vi "SSL Log Reader.vi"(10 "Cluster 2":refnum<vi>, 11 "Cluster":T1={"file path (use dialog)"=path "E:/Media/2016-07-01_cmdragons_immortals.log", "size (in bytes)"=0, "offset (in bytes)"=0, "Slide"=0.0, "Play"=FALSE, "Time Stamp"=timestamp(0 s since 1904-01-01), "Playing"=FALSE} {"Time Stamp" format="%<%.3X %x>T"; "Slide" min=0 max=1 scale=0.0..1.0; "offset (in bytes)" format="%.3p"; "size (in bytes)" format="%.3p"}) -> (0 "error out":errorcluster, 1 "Cluster 3":T1={"file path (use dialog)"=path "E:/Media/2016-07-01_cmdragons_immortals.log", "size (in bytes)"=0, "offset (in bytes)"=0, "Slide"=0.0, "Play"=FALSE, "Time Stamp"=timestamp(0 s since 1904-01-01), "Playing"=FALSE} {"Time Stamp" format="%<%.3X %x>T"; "Slide" min=0 max=1 scale=0.0..1.0; "offset (in bytes)" format="%.3p"; "size (in bytes)" format="%.3p"}, 2 "channel 2":T2, 3 "Channel out":T2)   [LabVIEW 2017]
uses:
  <extravilib>/ChannelInstances/Stream-a[.](u8).lvlib
  <extravilib>/ChannelInstances/Stream-a[.](u8)/)Channel.ctl
  Control/File Player.ctl
panel:
  out "error out 2":errorcluster
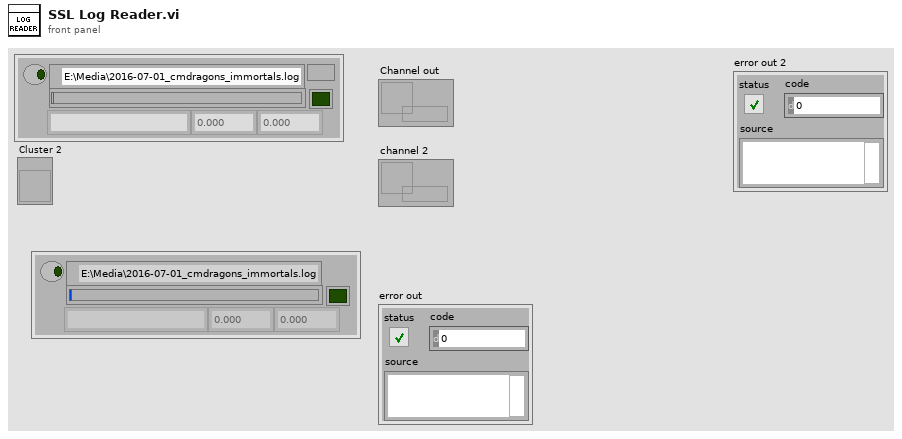
[diagram p1: front panel]
types:
  T1 = typedef "File Player.ctl" = cluster{"file path (use dialog)":path, "size (in bytes)":i64, "offset (in bytes)":i64, "Slide":sgl, "Play":bool, "Time Stamp":timestamp, "Playing":bool}
  T2 = typedef "Stream-a[.](u8).lvlib/)Channel.ctl" = refnum<queue>
  T3 = enum16{"open", "replace", "create", "open or create", "replace or create", "replace or create with confirmation"}
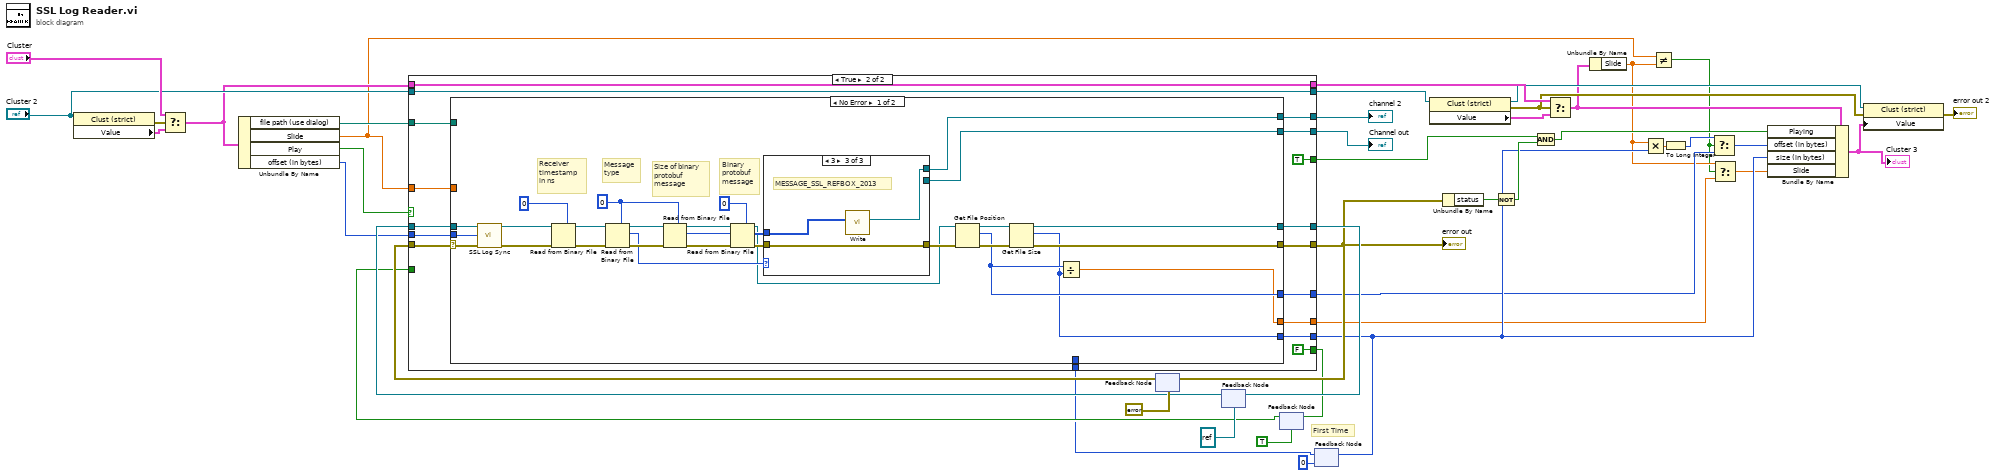
[diagram p0: block diagram]
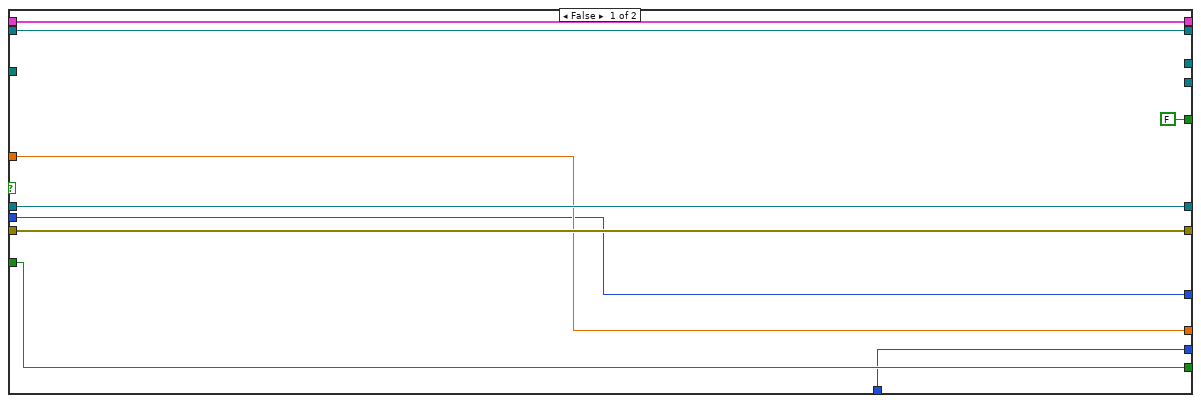
[diagram p2: hidden frame]
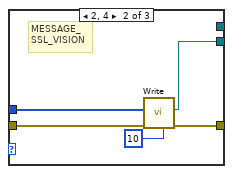
[diagram p4: hidden frame]
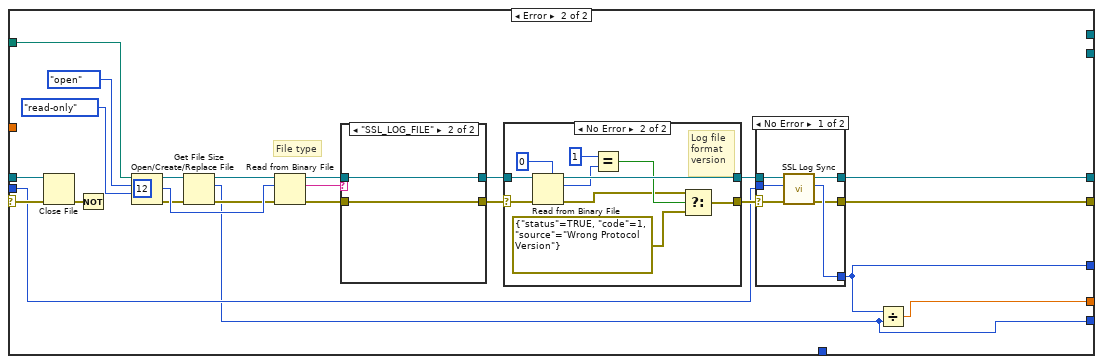
[diagram p5: hidden frame]
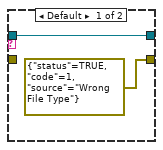
[diagram p7: hidden frame]
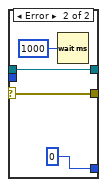
[diagram p8: hidden frame]
diagram:
  # "First Time"
  n1 = property on="Property Node" class="Clust (strict)"(reference="Cluster 2") -> (error out=w28:errorcluster, "Value"=w26:T1)  [unwired: 1 in, 1 out]
  n2 = Select(t="Cluster", s=w28, f=w26) -> (s? t:f=w19:T1)
  n3 = Unbundle By Name(w19) -> ("file path (use dialog)"=w25:path, "Slide"=w10:sgl, "Play"=w24:bool, "offset (in bytes)"=w13:i64)
  n4 = feedback #1(errorcluster {"status"=FALSE, "code"=0, "source"=""} ("error out")) -> (w39:errorcluster)
  n5 = feedback #2(refnum<file> refnum ("refnum out")) -> (w37:refnum<file>)
  n6 = feedback #3(TRUE) -> (w33:bool)
  n7 = feedback #4(i64 0 ("size (in bytes)")) -> (w30:i64)
  n8 = case shown="True" w24 {
    tunnel: [w44 w69] -> w7
    tunnel: w25 -> [_ w68]
    tunnel: [_ w67] -> w43
    tunnel: [_ w66] -> w42
    tunnel: w10 -> [w45 w63]
    tunnel: [w51 w65] -> w36
    tunnel: w39 -> [w51 w61]
    tunnel: [w52 w64] -> w38
    tunnel: w37 -> [w52 w62]
    tunnel: [w50 FALSE] -> w34
    tunnel: w33 -> [w50 _]
    tunnel: [w49 w59] -> w9
    tunnel: w30 -> [w49 w58]
    tunnel: [FALSE TRUE] -> w29
    tunnel: [w47 w56] -> w22
    tunnel: "Cluster 2" -> [w47 w56]
    tunnel: [w46 w55] -> w20
    tunnel: w19 -> [w46 w55]
    tunnel: [w45 w54] -> w2
    tunnel: w13 -> [w44 w53]
    frame False {
    }
    frame True {
      n9 = case shown="No Error" w61 {
        selector: w61 -> [w83 w113]
        tunnel: [w74 w116] -> w65
        tunnel: [w98 _] -> w66
        tunnel: [w97 _] -> w67
        tunnel: w68 -> [_ w123]
        tunnel: [w73 w110] -> w69
        tunnel: [w75 w114] -> w64
        tunnel: w62 -> [w82 w112]
        tunnel: w63 -> [_ _]
        tunnel: [w70 w107] -> w59
        tunnel: w58 -> [_ _]
        tunnel: [w72 w109] -> w54
        tunnel: w53 -> [w71 w108]
        frame No Error {
          w88 = 0 ("data type")
          # "Binary\nprotobuf\nmessage"
          # "Size of binary\nprotobuf \nmessage"
          # "Receiver \ntimestamp \nin ns"
          # "Message\ntype"
          n10 = call "SSL Log Sync.vi"("error in (no error)"=w83, "Slide"=w71, "Byte Stream File in"=w82) -> ("error out"=w78:errorcluster, "Byte Stream File out"=w79:refnum<file>)  [unwired: 6 in, 1 out]
          n11 = Read from Binary File(5:i64 0 ("data type"), 8:w78, 11:w79) -> (0:w93:errorcluster, 3:w94:refnum<file>)  [unwired: 3 in, 2 out]
          n12 = Read from Binary File(5:w88, 8:w93, 11:w94) -> (0:w90:errorcluster, 2:w84:i32, 3:w92:refnum<file>)  [unwired: 3 in, 1 out]
          n13 = Read from Binary File(5:w88, 8:w90, 11:w92) -> (0:w89:errorcluster, 2:w85:i32, 3:w91:refnum<file>)  [unwired: 3 in, 1 out]
          n14 = Read from Binary File(5:u8 0 ("data type"), 8:w89, 10:w85, 11:w91) -> (0:w86:errorcluster, 2:w87:u8[], 3:w80:refnum<file>)  [unwired: 2 in, 1 out]
          n15 = case shown="3" w84 {
            tunnel: w87 -> [_ w103 w105]
            tunnel: w86 -> [w99 w102 w106]
            tunnel: [w99 w102 w106] -> w81
            tunnel: [_ _ w104] -> w98
            tunnel: [_ w100 _] -> w97
            frame Default {
            }
            frame 2, 4 {
              # "MESSAGE_\nSSL_VISION"
              n16 = call <extravilib>:"Write.vi"("size (unlimited)"=10, "element"=w103) -> ("channel"=w100:T2)  [unwired: 7 in, 2 out]
            }
            frame 3 {
              # "MESSAGE_SSL_REFBOX_2013"
              n17 = call <extravilib>:"Write.vi"("element"=w105) -> ("channel"=w104:T2)  [unwired: 8 in, 2 out]
            }
          }
          n18 = Get File Position(4:w81, 7:w80) -> (0:w77:errorcluster, 2:w73:i64, 3:w76:refnum<file>)
          n19 = Get File Size(file=w76, error in=w77) -> (refnum out=w75:refnum<file>, size (in bytes)=w70:i64, 0:w74:errorcluster)
          n20 = Divide(x=w73, y=w70) -> (x/y=w72:dbl)
        }
        frame Error {
          # "File type"
          n21 = Close File(refnum=w112, error in=w113) -> (error out=w111:errorcluster)  [unwired: 1 out]
          n22 = Not(x=w111) -> ()  [unwired: 1 out]
          n23 = Open/Create/Replace File(file path (use dialog)=w123, operation (0:open)=T3."open", access (0:read/write)=enum16{"read/write", "read-only", "write-only"}."read-only") -> (refnum out=w127:refnum<file>, error out=w124:errorcluster)  [unwired: 3 in, 1 out]
          n24 = Get File Size(file=w127, error in=w124) -> (refnum out=w126:refnum<file>, size (in bytes)=w107:i64, 0:w125:errorcluster)
          n25 = Read from Binary File(8:w125, 10:12 ("count (1)"), 11:w126) -> (0:w121:errorcluster, 2:w122:string, 3:w118:refnum<file>)  [unwired: 3 in, 1 out]
          n26 = case shown="\"SSL_LOG_FILE\"" w122 {
            tunnel: w121 -> [_ w146]
            tunnel: [errorcluster {"status"=TRUE, "code"=1, "source"="Wrong File Type"} ("error out") w146] -> w120
            tunnel: [w143 w145] -> w119
            tunnel: w118 -> [w143 w145]
            frame Default {
            }
            frame "SSL_LOG_FILE" {
            }
          }
          n27 = case shown="No Error" w120 {
            selector: w120 -> [w132 w141]
            tunnel: [w132 w136] -> w117
            tunnel: w119 -> [w131 w140]
            tunnel: [w131 w139] -> w115
            frame Error {
            }
            frame No Error {
              # "Log file \nformat \nversion"
              n28 = Read from Binary File(5:0 ("prompt (Open existing file)"), 8:w141, 11:w140) -> (0:w134:errorcluster, 2:w138:i32, 3:w139:refnum<file>)  [unwired: 3 in, 1 out]
              n29 = Equal?(x=1, y=w138) -> (x = y?=w135:bool)
              n30 = Select(t=w134, s=w135, f=errorcluster {"status"=TRUE, "code"=1, "source"="Wrong Protocol Version"} ("error out")) -> (s? t:f=w136:errorcluster)
            }
          }
          n31 = case shown="No Error" w117 {
            selector: w117 -> [w152 w156]
            tunnel: [w148 w156] -> w116
            tunnel: w115 -> [w151 w155]
            tunnel: [w150 w155] -> w114
            tunnel: [w149 i64 0 ("offset (in bytes)")] -> w110
            tunnel: w108 -> [w147 _]
            frame No Error {
              n32 = call "SSL Log Sync.vi"("error in (no error)"=w152, "Slide"=w147, "Byte Stream File in"=w151) -> ("error out"=w148:errorcluster, "Offset"=w149:i64, "Byte Stream File out"=w150:refnum<file>)  [unwired: 6 in]
            }
            frame Error {
              n33 = Wait (ms)(milliseconds to wait=u32 1000) -> ()  [unwired: 1 out]
            }
          }
          n34 = Divide(x=w110, y=w107) -> (x/y=w109:dbl)
        }
      }
    }
  }
  "Channel out" <- w43
  "channel 2" <- w42
  "error out" <- w36
  n35 = feedback-in #1(w36) -> ()
  n36 = feedback-in #2(w38) -> ()
  n37 = feedback-in #3(w34) -> ()
  n38 = feedback-in #4(w9) -> ()
  n39 = property on="Property Node" class="Clust (strict)"(reference=w22) -> (reference out=w16:refnum<vi>, error out=w15:errorcluster, "Value"=w23:T1)  [unwired: 1 in]
  n40 = Unbundle By Name(w36) -> ("status"=w41:bool)
  n41 = Not(x=w41) -> (.not. x?=w17:bool)
  n42 = And(x=w29, y=w17) -> (x .and. y?=w18:bool)
  n43 = Select(t=w20, s=w15, f=w23) -> (s? t:f=w11:T1)
  n44 = Unbundle By Name(w11) -> ("Slide"=w3:sgl)
  n45 = Multiply(x=w3, y=w9) -> (x*y=w5:sgl)
  n46 = Not Equal?(x=w10, y=w3) -> (x != y?=w1:bool)
  n47 = To Long Integer(number=w5) -> (32bit integer=w6:i32)
  n48 = Select(t=w6, s=w1, f=w7) -> (s? t:f=w8:i64)
  n49 = Select(t=w3, s=w1, f=w2) -> (s? t:f=w4:dbl)
  n50 = Bundle By Name(cluster=w11, "Playing"=w18, "offset (in bytes)"=w8, "size (in bytes)"=w9, "Slide"=w4) -> (w12:T1)
  "Cluster 3" <- w12
  n51 = property on="Property Node" class="Clust (strict)"(reference=w16, error in=w15, "Value"=w12) -> (error out=→"error out 2":errorcluster)  [unwired: 1 out]
